vi "Get LabVIEW Install Paths.vi"(8 "Error In":errorcluster) -> (0 "Error Out":errorcluster, 2 "Path":path[](array[path]), 3 "Version":string[](array[string]))   [LabVIEW 2011, in "LVH-Toolbox.lvlib" / "LVH-SystemTools.lvlib"]
uses:
  LVH-SystemTools.lvlib
  <vilib>/registry/registry.llb/Read Registry Value Simple STR.vi
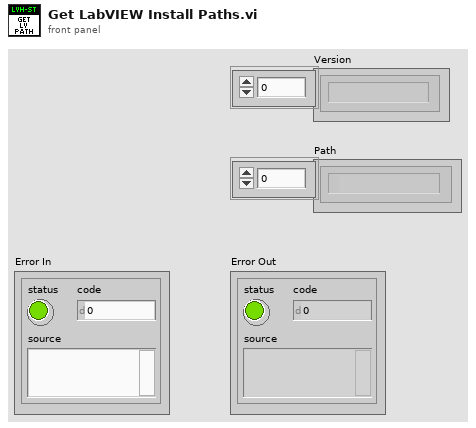
[diagram p1: front panel]
types:
  T1 = typedef "Registry refnum.ctl" = refnum<k1>
  T2 = cluster{"numSubKeys":i32, "maxSubKeyLen":i32, "maxSubKeyClassLen":i32}
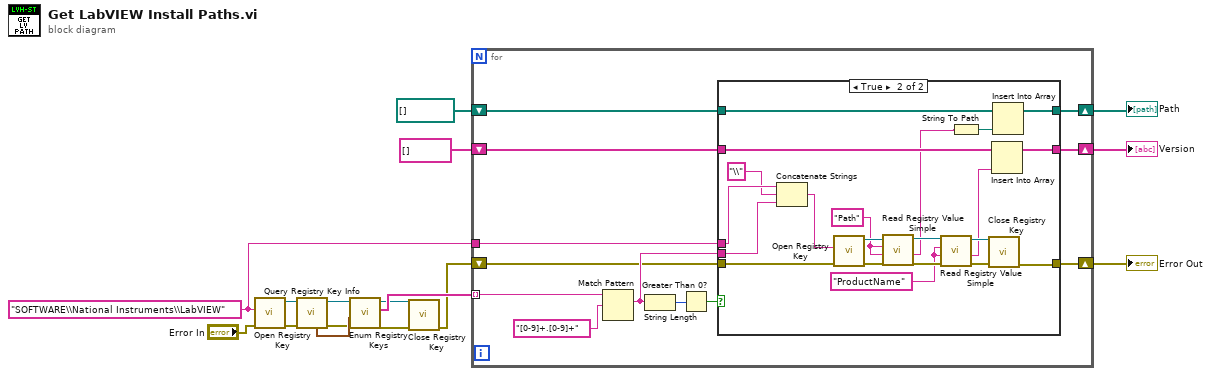
[diagram p0: block diagram]
diagram:
  w8 = "SOFTWARE\\National Instruments\\LabVIEW" ("subkey")
  n1 = call <vilib>:"Open Registry Key.vi"("error in (no error)"="Error In", "subkey"=w8) -> ("error out"=w13:errorcluster, "refnum out"=w16:T1)  [unwired: 8 in]
  n2 = call <vilib>:"Query Registry Key Info.vi"("error in (no error)"=w13, "refnum"=w16) -> ("error out"=w12:errorcluster, "refnum out"=w15:T1, "subkey info"=w14:T2)  [unwired: 5 in, 2 out]
  n3 = call <vilib>:"Enum Registry Keys.vi"("error in (no error)"=w12, "subkey info"=w14, "refnum"=w15) -> ("error out"=w9:errorcluster, "subkeys"=w11:string[], "refnum out"=w10:T1)  [unwired: 6 in]
  n4 = call <vilib>:"Close Registry Key.vi"("error in (no error)"=w9, "refnum"=w10) -> ("error out"=w7:errorcluster)  [unwired: 5 in]
  n5 = for {
    tunnel: w11 -> [w28] mode=indexing
    tunnel: w8 -> [w24]
    shift-right: [w21] -> w5
    shift-left: w7 -> [w22]
    shift-right: [w19] -> w3
    shift-left: string[] [] -> [w20]
    shift-right: [w17] -> w1
    shift-left: path[] [] -> [w18]
    n6 = Match Pattern(string=w28, regular expression="[0-9]+.[0-9]+") -> (match substring=w23:string)  [unwired: 1 in, 3 out]
    n7 = String Length(string=w23) -> (length=w26:i32)
    n8 = Greater Than 0?(x=w26) -> (x > 0?=w25:bool)
    n9 = case shown="True" w25 {
      tunnel: w24 -> [_ w52]
      tunnel: w23 -> [_ w48]
      tunnel: w22 -> [w31 w50]
      tunnel: [w31 w44] -> w21
      tunnel: w20 -> [w29 w38]
      tunnel: [w29 w36] -> w19
      tunnel: w18 -> [w30 w35]
      tunnel: [w30 w34] -> w17
      frame False {
      }
      frame True {
        w39 = "ProductName" ("value")
        w45 = "Path" ("value")
        n10 = Concatenate Strings(w52, "\\" ("string"), w48) -> (w51:string)
        n11 = call <vilib>:"Open Registry Key.vi"("error in (no error)"=w50, "subkey"=w51) -> ("error out"=w46:errorcluster, "refnum out"=w47:T1)  [unwired: 8 in]
        n12 = call-poly <vilib>:"Read Registry Value Simple.vi"("error in (no error)"=w46, "default data"=w45, "value"=w45, "refnum"=w47) -> ("error out"=w42:errorcluster, "String/Binary data"=w33:string, "refnum out"=w41:T1)  [unwired: 2 in, 1 out]
        n13 = call-poly <vilib>:"Read Registry Value Simple.vi"("error in (no error)"=w42, "default data"=w39, "value"=w39, "refnum"=w41) -> ("error out"=w43:errorcluster, "String/Binary data"=w37:string, "refnum out"=w40:T1)  [unwired: 2 in, 1 out]
        n14 = String To Path(string=w33) -> (path=w32:path)
        n15 = call <vilib>:"Close Registry Key.vi"("error in (no error)"=w43, "refnum"=w40) -> ("error out"=w44:errorcluster)  [unwired: 5 in]
        n16 = Insert Into Array(array=w38, new element=w37) -> (w36:string[])  [unwired: 1 in]
        n17 = Insert Into Array(array=w35, new element=w32) -> (w34:path[])  [unwired: 1 in]
      }
    }
  }
  "Error Out" <- w5
  "Version" <- w3
  "Path" <- w1
